vi "Gradient Estimation Plot.vi"(8 "error in":errorcluster, 10 "Image":T1, 11 "Pixel Column Number from edge detection":i32) -> (0 "error out":errorcluster, 3 "Value of Pixel at which maximum gradient occurs":i32)   [LabVIEW 2016]
uses:
  <vilib>/vision/Image Controls.llb/IMAQ Image.ctl
  <vilib>/vision/NI_Vision_Development_Module.lvlib
panel:
  out "Pixel vs Intensity Graph":cluster{"Y":dbl[], "Y":dbl[]}[](graph)
  out "Pixel vs Gradient Graph":cluster{"Y":dbl[], "Y":dbl[]}[](graph)
  out "Maximum Gradient":u8
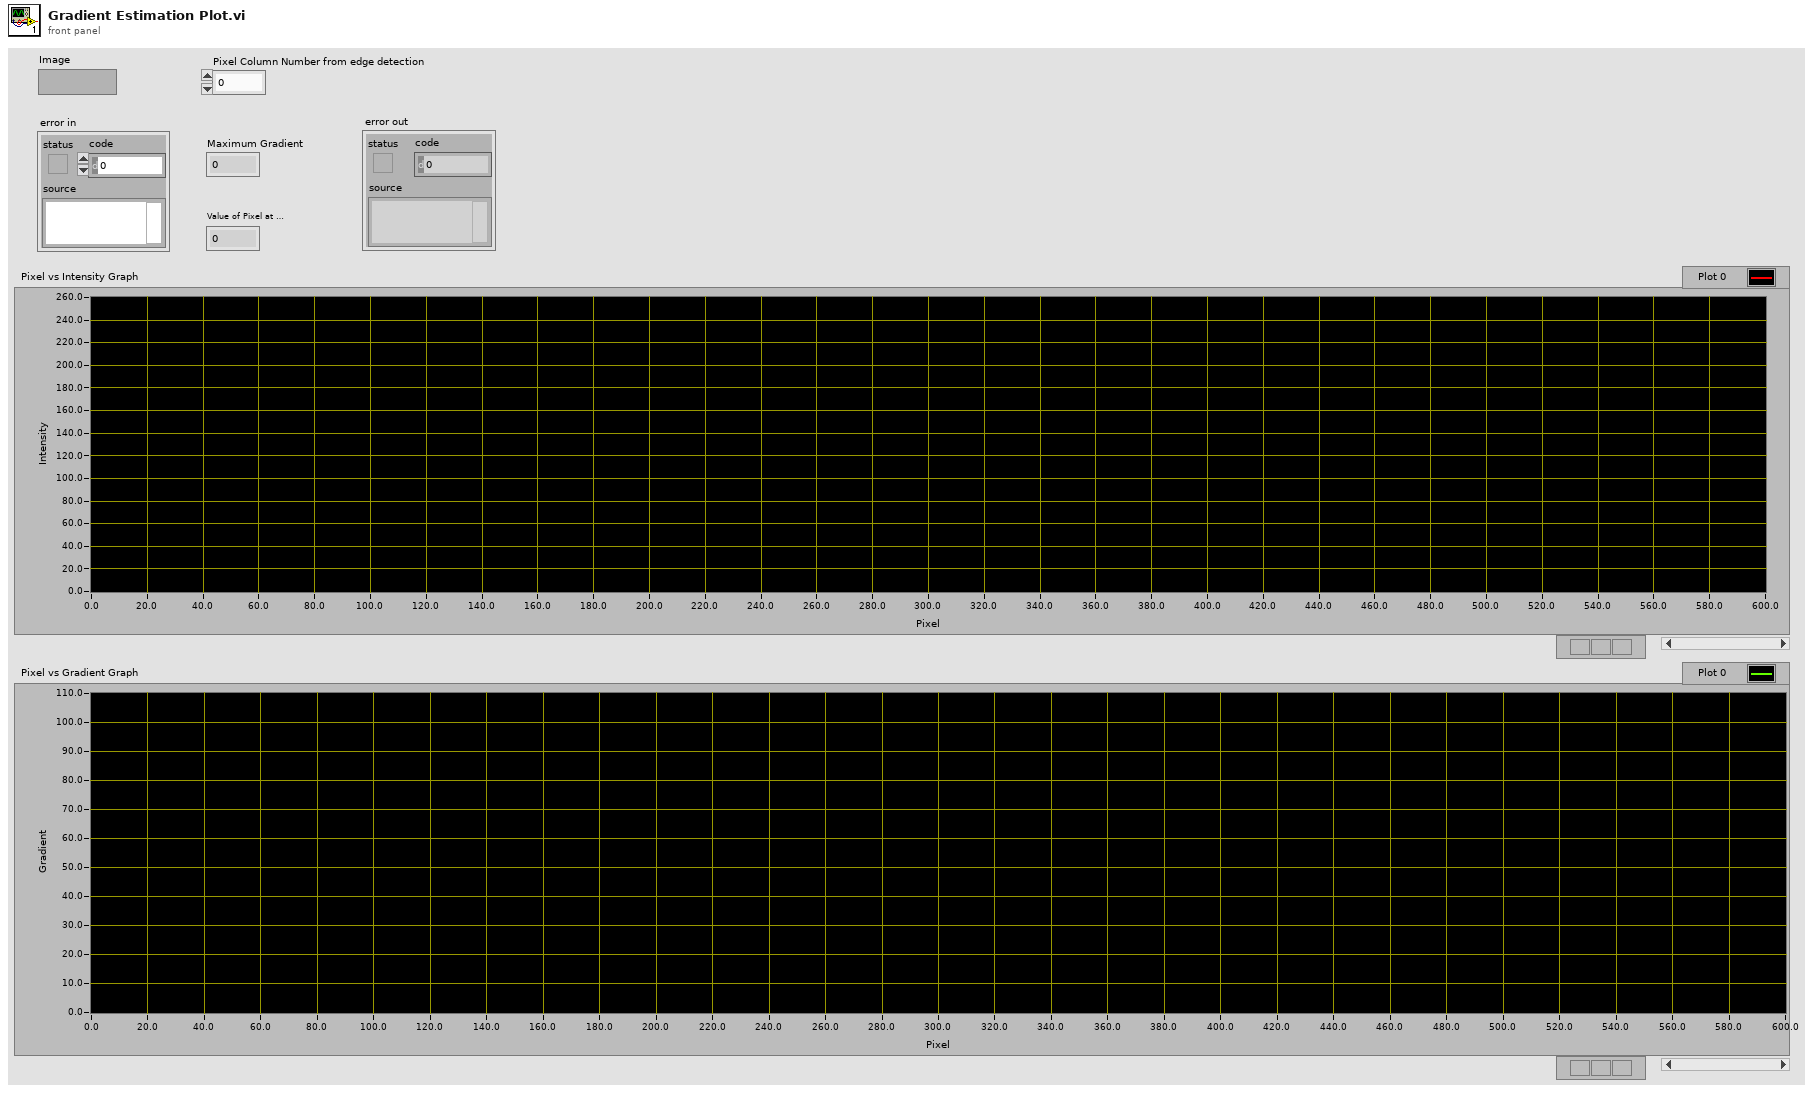
[diagram p1: front panel]
types:
  T1 = typedef "IMAQ Image.ctl" = refnum<image>
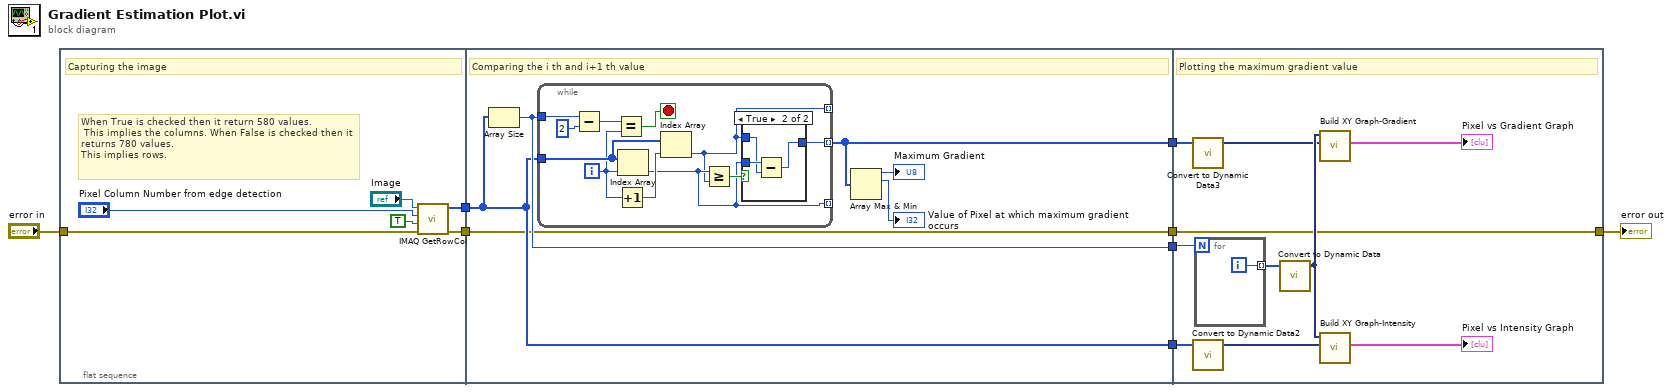
[diagram p0: block diagram]
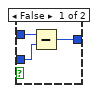
[diagram p2: hidden frame]
diagram:
  n1 = flat-sequence {
    tunnel: [w12] -> w8
    tunnel: "error in" -> [w10]
    tunnel: [w9] -> w3
    tunnel: [w20] -> w7
    tunnel: [w19] -> w6
    tunnel: w8 -> [w19]
    tunnel: [w18] -> w5
    tunnel: w3 -> [w15]
    tunnel: [w15] -> w2
    tunnel: w7 -> [w44]
    tunnel: w6 -> [w45]
    tunnel: w5 -> [w40]
    tunnel: w2 -> [w38]
    tunnel: [w38] -> w1
    frame #0 {
      # "When True is checked then it return 580 values.\n This implies the columns. When False is checked then it returns 780 values. \nThis implies rows."
      # "Capturing the image"
      n2 = call "IMAQ GetRowCol"("Image"="Image", "Number"="Pixel Column Number from edge detection", "Row / Column (Row)"=TRUE, "error in (no error)"=w10) -> ("Pixels (U8)"=w12:u8[], "error out"=w9:errorcluster)  [unwired: 2 in, 3 out]
    }
    frame #1 {
      # "Comparing the i th and i+1 th value"
      n3 = Array Size(array=w19) -> (size(s)=w20:i32)
      n4 = while {
        tunnel: w20 -> [w27]
        tunnel: w19 -> [w29]
        tunnel: [w22] -> _ mode=indexing
        tunnel: [w23] -> _ mode=indexing
        tunnel: [w21] -> w18 mode=indexing
        i -> [w28]
        stop <- w31 stop-if-true
        n5 = Subtract(x=w27, y=2 ("Number")) -> (x-y=w25:i32)
        n6 = Equal?(x=w25, y=w28) -> (x = y?=w31:bool)
        n7 = Increment(x=w28) -> (x+1=w30:i32)
        n8 = Index Array(array=w29, index=w28) -> (element=w23:u8)
        n9 = Index Array(array=w29, index=w30) -> (element=w22:u8)
        n10 = Greater Or Equal?(x=w23, y=w22) -> (x >= y?=w24:bool)
        n11 = case shown="True" w24 {
          tunnel: w23 -> [w33 w37]
          tunnel: w22 -> [w34 w36]
          tunnel: [w32 w35] -> w21
          frame False {
            n12 = Subtract(x=w34, y=w33) -> (x-y=w32:u8)
          }
          frame True {
            n13 = Subtract(x=w37, y=w36) -> (x-y=w35:u8)
          }
        }
      }
      n14 = Array Max & Min(array=w18) -> (max value=→"Maximum Gradient":u8, max index (indices)=→"Value of Pixel at which maximum gradient occurs":i32)  [unwired: 2 out]
    }
    frame #2 {
      # "Plotting the maximum gradient value"
      n15 = call "Convert to Dynamic Data3"("Array"=w40) -> ("Dynamic Data Type"=w42:dynamicdata)  [unwired: 3 in]
      n16 = call "Convert to Dynamic Data2"("Array"=w45) -> ("Dynamic Data Type"=w47:dynamicdata)  [unwired: 3 in]
      n17 = for {
        N: w44 -> [_]
        tunnel: [w48] -> w46 mode=indexing
        i -> [w48]
      }
      n18 = call "Convert to Dynamic Data"("Array"=w46) -> ("Dynamic Data Type"=w43:dynamicdata)  [unwired: 3 in]
      n19 = call "Build XY Graph-Gradient"("Y Input"=w42, "X Input"=w43) -> ("XY Graph"=→"Pixel vs Gradient Graph":cluster{"X":dbl[], "Y":dbl[]}[])  [unwired: 8 in, 1 out]
      n20 = call "Build XY Graph-Intensity"("Y Input"=w47, "X Input"=w43) -> ("XY Graph"=→"Pixel vs Intensity Graph":cluster{"X":dbl[], "Y":dbl[]}[])  [unwired: 8 in, 1 out]
    }
  }
  "error out" <- w1
